vi "Main.vi"() -> ()   [LabVIEW 2017]
doc: "Use this template to build a simple state machine design pattern. Each state executes code and determines which state to transition to."
uses:
  <vilib>/robotics/Controls/Compass Indicator/Compass Indicator.xctl
  controls/State.ctl
  controls/Data.ctl
  <vilib>/Instr/_visa.llb/VISA Configure Serial Port (Instr).vi
  support/VariaveisGlobais.vi
panel:
  out "DadosGPS":dbl[][](array[numeric])
  in  "Controles":T1(tab)
  out "Corrente de Saída":dbl caption="Numeric"
  out "SOC":dbl(slide)=100.0 scale=0.0..100.0
  out "Volt(V)":dbl(knob)=54.0 caption="Gauge" scale=0.0..60.0
  out "Velocidade do Barco":dbl(knob)=30.0 caption="Gauge" scale=0.0..50.0
  out "Corrente de Entrada":dbl caption="Numeric"
  out "Longitude do Barco":dbl=-48.640396 format="%#.6g"
  out "Banco de Bateria":dbl[][](array[slide])=[[3.33, 3.33, 3.33, 3.33], [3.33, 3.33, 3.33, 3.33], [3.33, 3.33, 3.33, 3.33], [3.33, 3.33, 3.33, 3.33], [3.33, 3.33, 3.33, 3.33]] scale=0.0..5.0
  out "Voltagem Mínima":dbl=3.33
  out "Voltagem Máxima":dbl=3.33
  out "Sistema de Placa Solar":bool[][](array[boolean])
  in  "Color Box":u32(colorbox)=16777225
  out "Latitude do Barco":dbl=-26.244263 format="%#.6g"
  out "Latitude do Terra":dbl=-26.244263 format="%#.6g"
  out "Longitude do Terra":dbl=-48.640396 format="%#.6g"
  out "Compass Indicator":dbl(xcontrol)
  out "Distance to Destination km":dbl=0.005416306273989337
  out "Dados Recebidos":string
  out "PlotGeral":dbl[][](graph)
  out "Plotagem":dbl[](graph)
  in  "PlotarDados":u16(ring) caption="Ring" items=["Voltagem", "CorrenteE", "CorrenteS", "Velocidade"]
  out "Historico de Dados":string[][](table)
  in  "Intercalar":i32=1
  in  "N° Pontos":i32=5
  in  "Adionar Pontos":bool
  in  "WebBrowser":refnum<k7>(container)
  in  "Color":string(combo)
  in  "Size":string(combo)
  in  "Character":string(combo)
  in  "Latitude 2":dbl=-3.091948 format="%#.6g"
  in  "Longitude 2":dbl=-60.017863 format="%#.6g"
  in  "Zoom":sgl=16.0 format="%#.1g"
  in  "Size Y":dbl=650.0
  in  "Size X":dbl=450.0
  in  "Map Format":string(combo)="roadmap"
  in  "AtualizarMapa":bool
  in  "Dados no Arquivo":bool
  in  "Titulo do Arquivo":string="Telemetria-"
  in  "Inserir Data":bool=TRUE
  in  "Salvar":bool
  in  "Abrir":bool
  in  "Baud Rate":string(combo)="115200"
  in  "Porta COM":refnum<visa-resource-name>="COM4"
  in  "Data Bits":u16=8 caption="Numeric"
  in  "Parity":enum16{"None", "Odd", "Even", "Mark", "Space"}(ring)
  in  "Conectar":bool
  in  "Desconectar":bool
  in  "ByteCount":u32=100 caption="Numeric"
  out "ProgressoBarco":dbl(slide) scale=0.0..1.0
  in  "DesligarApp":bool
  in  "ResetButton":bool
  in  "Janela":T2(radio)
  in  "Cancel":bool
  in  "LerDados":bool
  # "Telemetria - Leviatã"
  # "Cargas"
  # "Banco de Baterias"
  # "Poraquê"
  # "Plotagem de Dados"
  # "Análise de Localização no Mapa"
  # "Dados de Telemetria"
  # "Configuração de Porta"
  # "Leviatã: Barco Poraquê\ntime de telemetria do barco a fim de realizar a leitura da bateria do barco\n\n\n\n\n\n\n\n\n\nDesenvolvido por: Alan Shishido / Igor Souza"
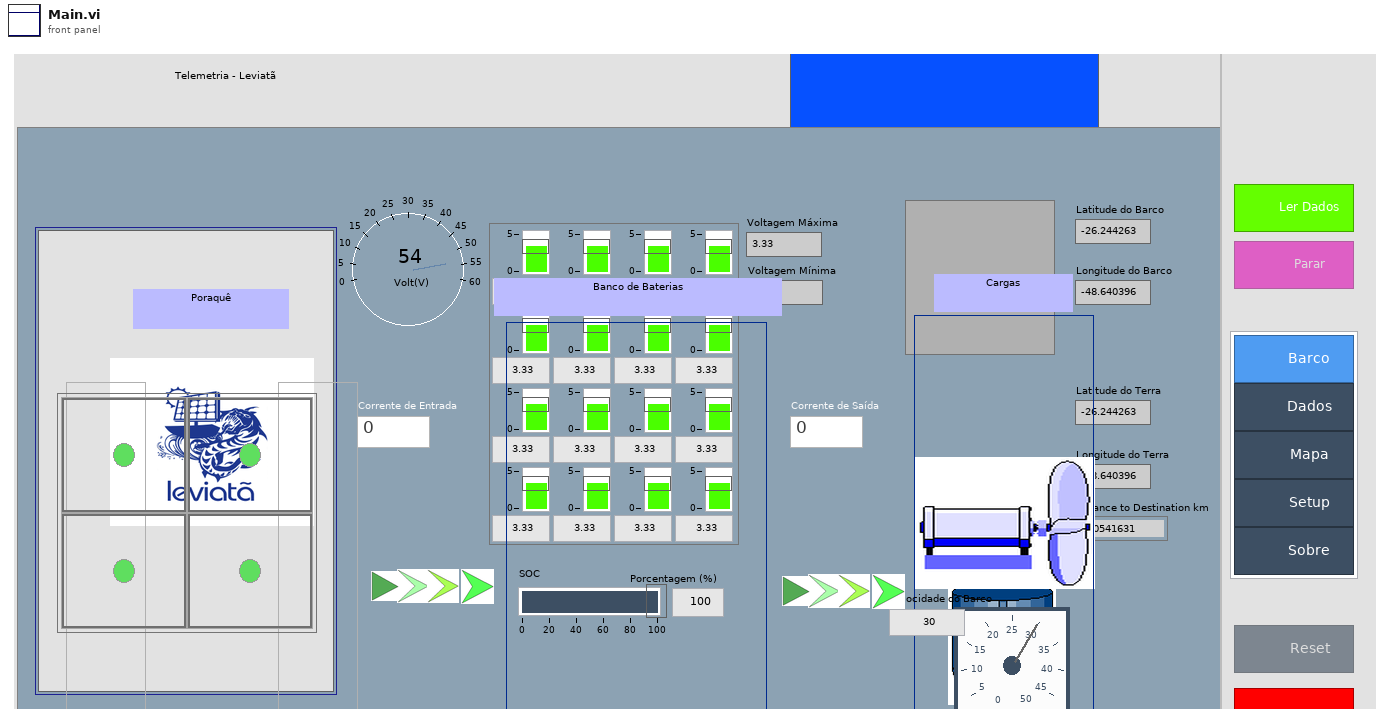
[diagram p1: front panel]
types:
  T1 = enum32{"Barco", "Gráfico", "Mapa", "Configuração", "Sobre"}
  T2 = enum32{"BarcoButton", "DadosButton", "MapaButton", "SetupButton", "SobreButton"}
  T3 = typedef "Data.ctl" = cluster{"PararOperação?":bool, "DadosSerial":string, "Dados 0":string, "Dados 1":string, "Dados 2":string, "Dados 3":string, "Dados 4":string, "Dados 5":string, "Dados 6":string, "Dados 7":string, "Dados 8":string, "Dados 9":string, "Dados 10":string, "Dados 11":string, "Dados 12":string, "Dados 13":string, "Dados 14":string, "Dados 15":string}
  T4 = cluster{"DadosBMS":T3, "SetupMapa":cluster{"Marker":string, "Path":string, "Markers Coordinates":string[][]}, "IteraçãoPrograma":cluster{"varBarco":i32, "varLerDados1":bool, "varLerDados2":bool, "varLerDados3":bool, "varLerDados4":bool}}
  T5 = typedef "State.ctl" = enum16{"Inicialização", "EsperaEvento", "bDesconectarSerial", "bConectar Serial", "bLerDadosSerial", "ProcessaDadosSerial", "AtualizaDadosSerial", "ArquivoDadosIncremental", "ClearAllDisplay", "AtualizarStaticMaps", "AdicionarPontosStaticMaps", "Sair"}
  T6 = enum8{"Enabled", "Disabled", "Disabled and Grayed Out"}
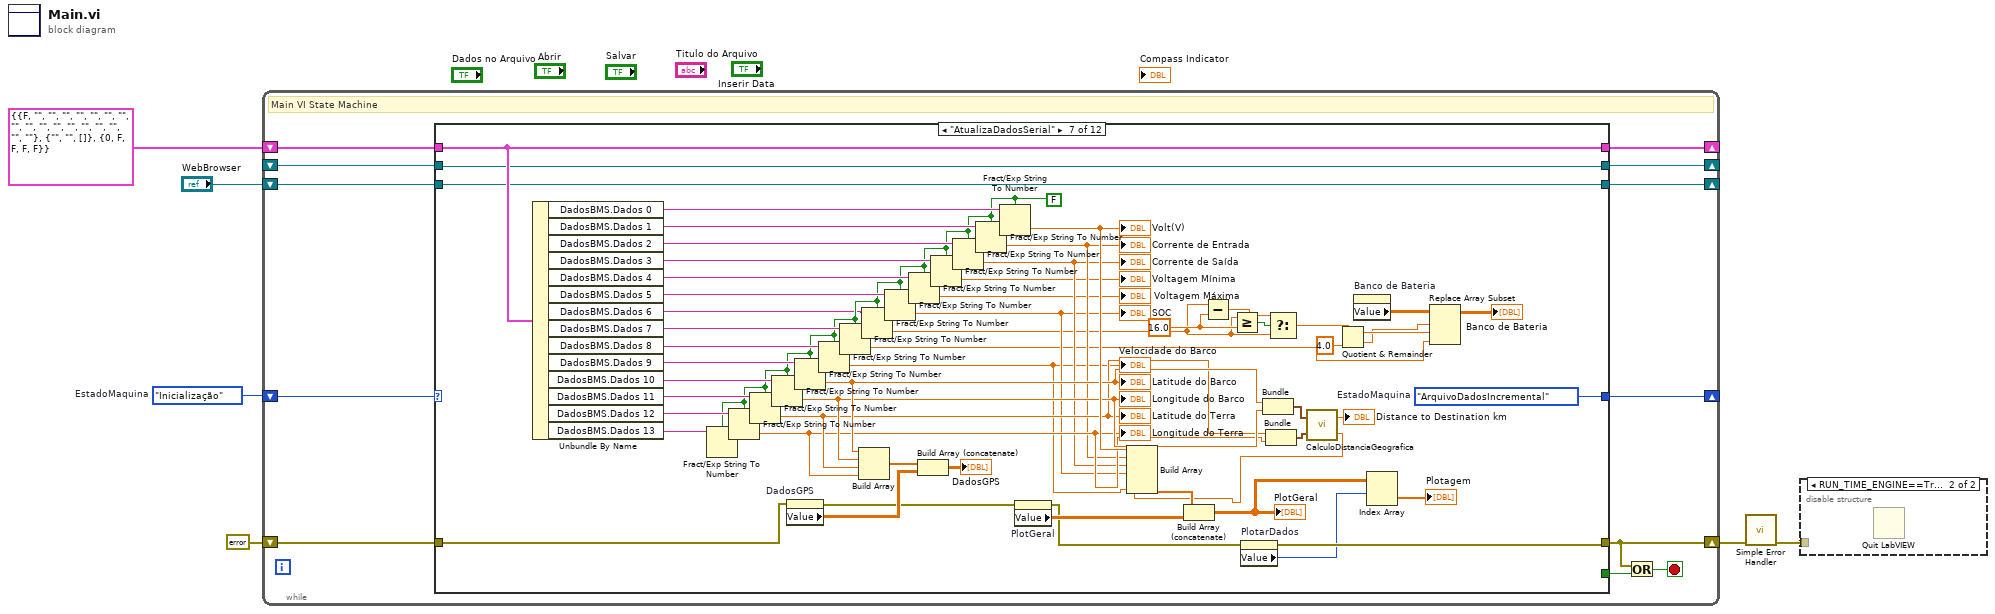
[diagram p0: block diagram]
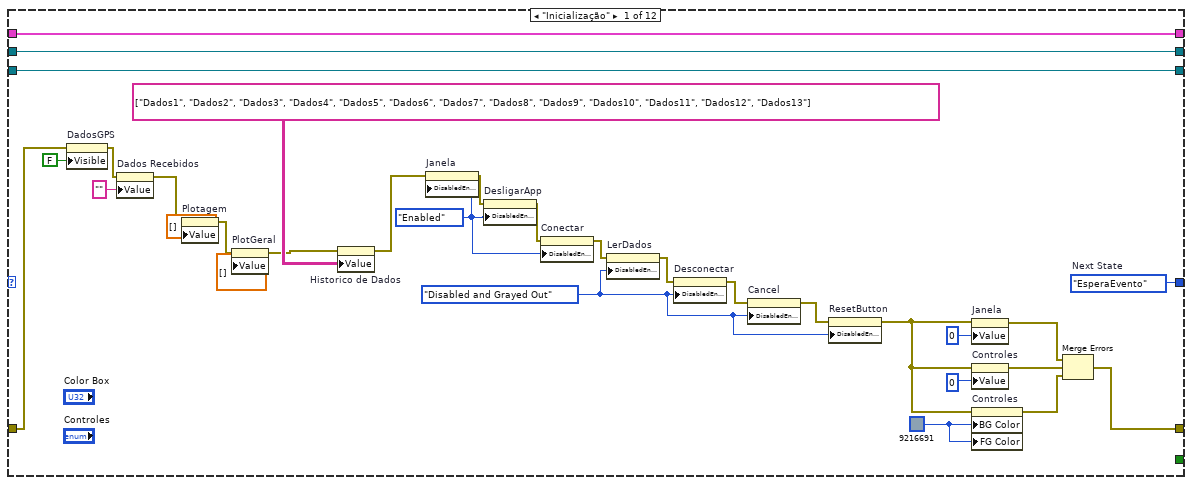
[diagram p2: hidden frame]
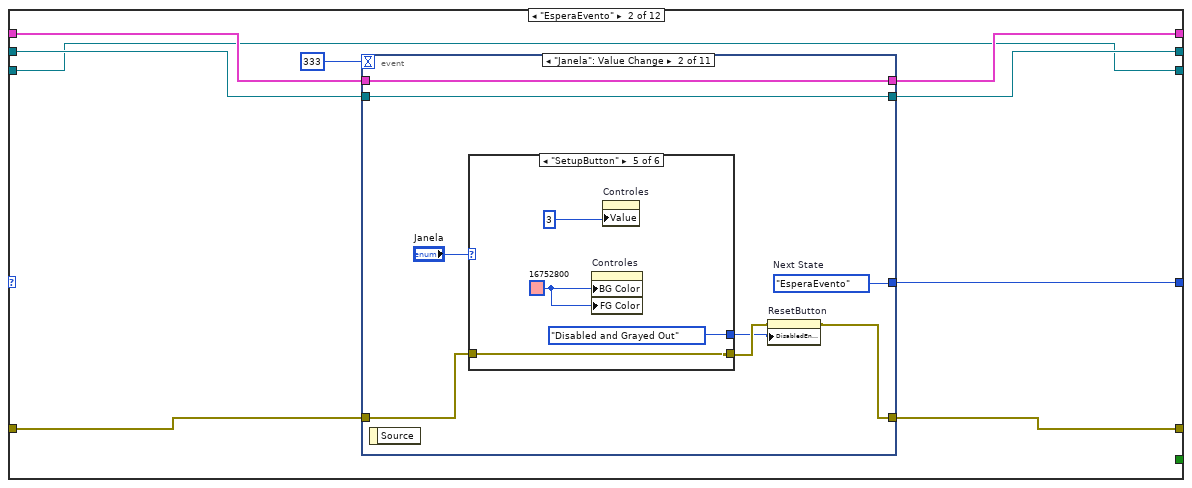
[diagram p3: hidden frame]
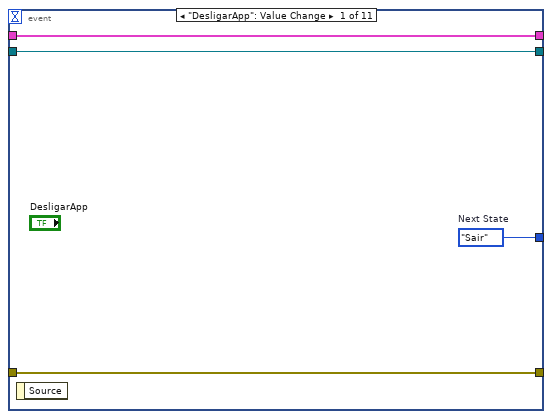
[diagram p4: hidden frame]
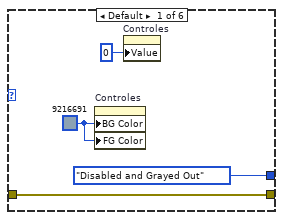
[diagram p5: hidden frame]
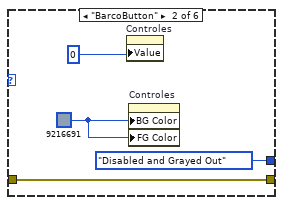
[diagram p6: hidden frame]
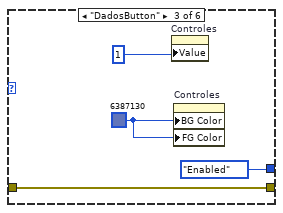
[diagram p7: hidden frame]
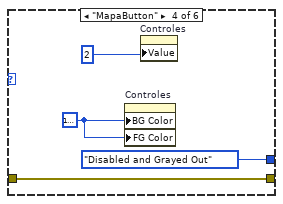
[diagram p8: hidden frame]
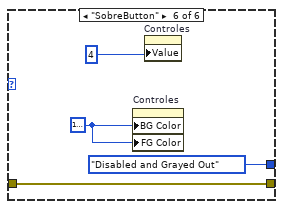
[diagram p9: hidden frame]
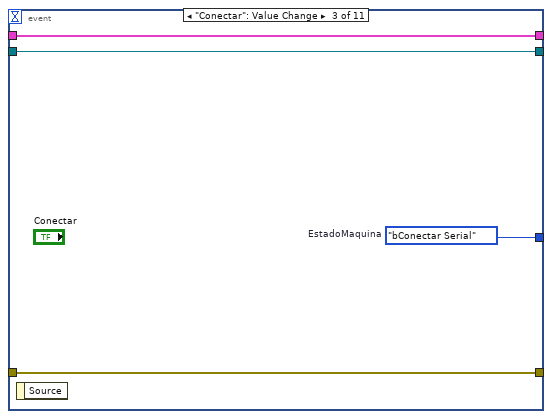
[diagram p10: hidden frame]
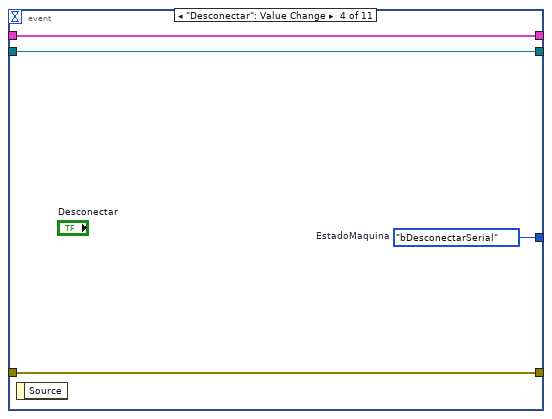
[diagram p11: hidden frame]
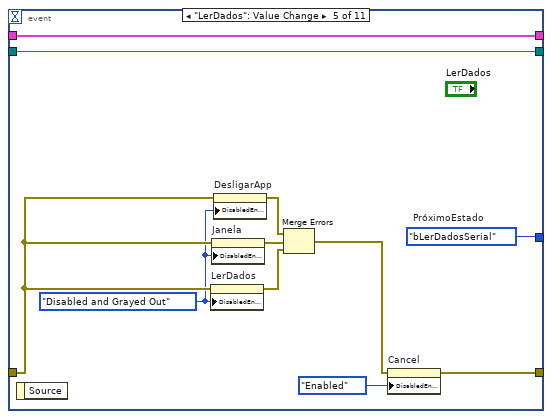
[diagram p12: hidden frame]
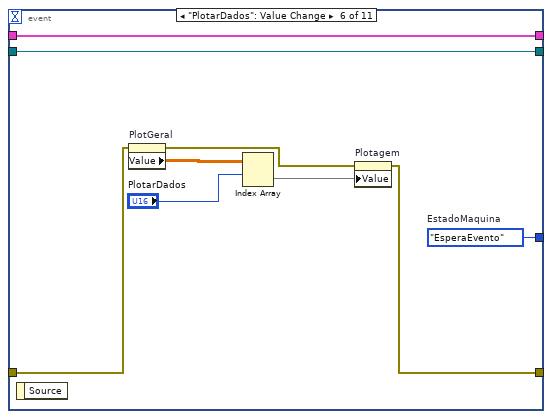
[diagram p13: hidden frame]
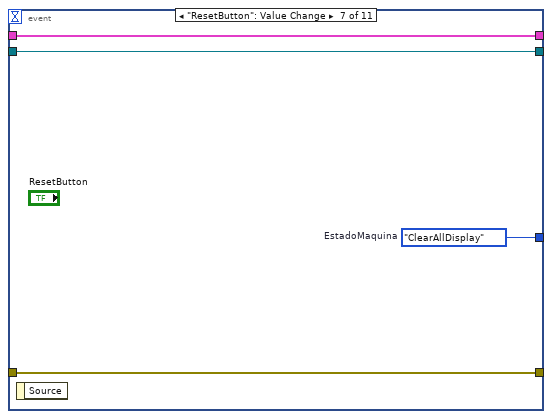
[diagram p14: hidden frame]
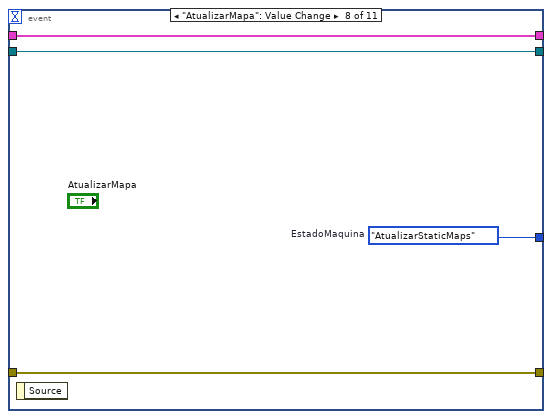
[diagram p15: hidden frame]
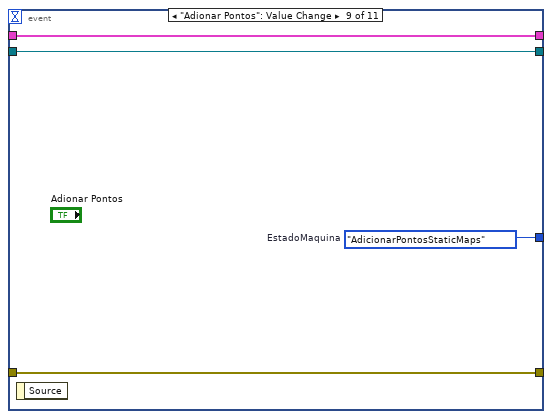
[diagram p16: hidden frame]
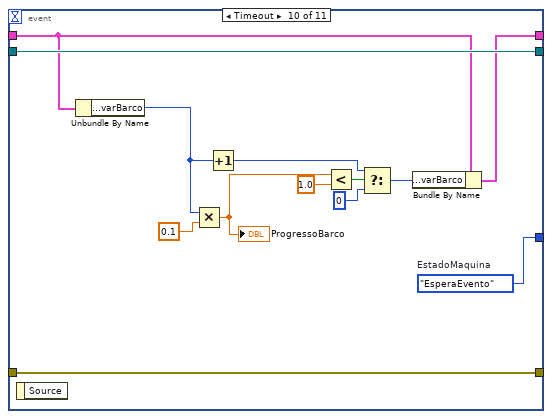
[diagram p17: hidden frame]
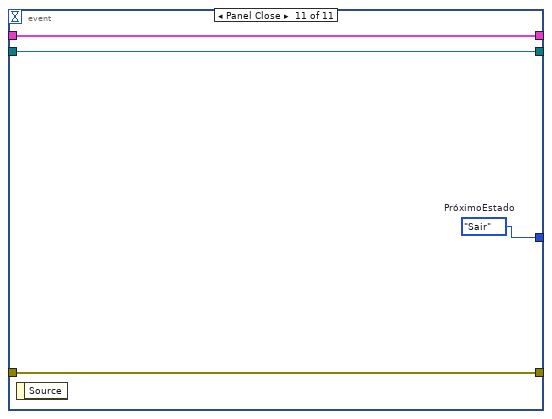
[diagram p18: hidden frame]
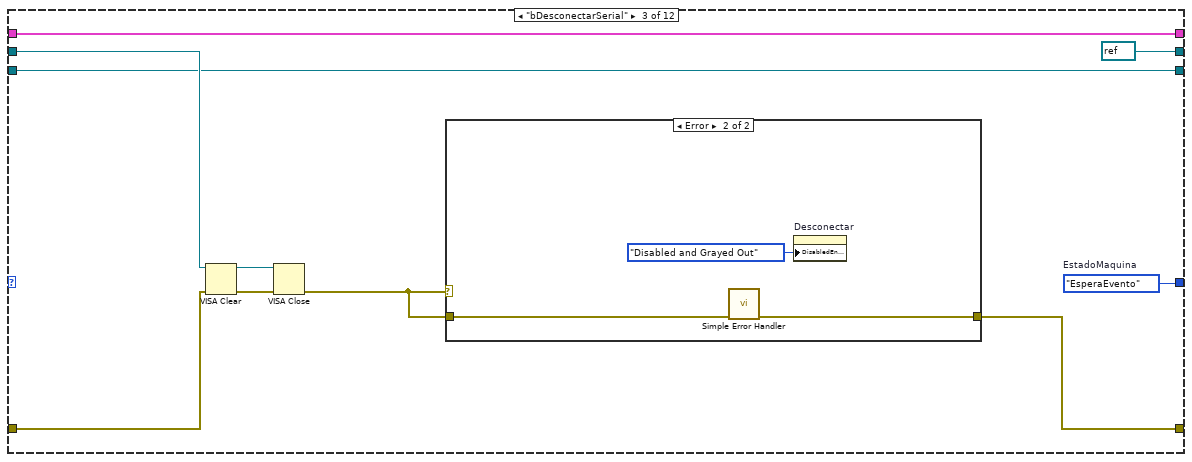
[diagram p19: hidden frame]
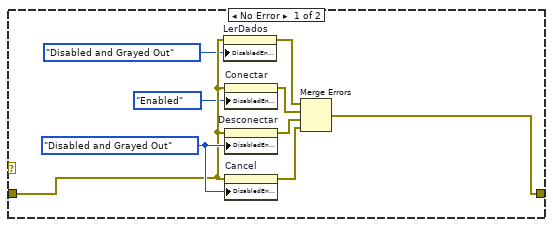
[diagram p20: hidden frame]
diagram:
  w6 = State."Inicialização"  # EstadoMaquina
  n1 = while {
    shift-right: [w17] -> _
    shift-left: w6 -> [w18]
    shift-right: [w15] -> _
    shift-left: T4 {"DadosBMS"={"PararOperação?"=FALSE, "DadosSerial"="", "Dados 0"="", "Dados 1"="", "Dados 2"="", "Dados 3"="", "Dados 4"="", "Dados 5"="", "Dados 6"="", "Dados 7"="", "Dados 8"="", "Dados 9"="", "Dados 10"="", "Dados 11"="", "Dados 12"="", "Dados 13"="", "Dados 14"="", "Dados 15"=""}, "SetupMapa"={"Marker"="", "Path"="", "Markers Coordinates"=[]}, "IteraçãoPrograma"={"varBarco"=0, "varLerDados1"=FALSE, "varLerDados2"=FALSE, "varLerDados3"=FALSE, "varLerDados4"=FALSE}} -> [w16]
    shift-right: [w11] -> w4
    shift-left: errorcluster {"status"=FALSE, "code"=0, "source"=""} ("error constant") -> [w14]
    shift-right: [w10] -> _
    shift-left: _ -> [w9]
    shift-right: [w7] -> _
    shift-left: "WebBrowser" -> [w8]
    stop <- w12 stop-if-true
    # "Main VI State Machine"
    n2 = case shown="\"AtualizaDadosSerial\"" w18 {
      tunnel: [w49 w58 w160 w191 w235 w273 w414 w455 w466 w490 w500 w535] -> w17
      tunnel: [_ _ _ _ _ _ _ _ _ _ _ w533] -> w13
      tunnel: w16 -> [w43 w57 w161 w192 w237 w268 w416 w421 w468 w479 w499 w534]
      tunnel: [w43 w56 w161 w192 w236 w267 w416 w420 w468 w479 w498 w534] -> w15
      tunnel: w14 -> [w26 w55 w158 w190 w238 w277 w386 w452 w458 w470 w502 w530]
      tunnel: [w32 w54 w155 w185 w222 w277 w384 w451 w457 w476 w502 errorcluster {"status"=FALSE, "code"=0, "source"=""} ("error constant")] -> w11
      tunnel: [w48 w52 refnum<visa-resource-name> refnum ("VISA resource name out") w184 w227 w276 w415 w418 w467 w491 w501 refnum<visa-resource-name> refnum ("VISA resource name out")] -> w10
      tunnel: w9 -> [w48 w51 w159 _ w239 w276 w415 w418 w467 w491 w501 w532]
      tunnel: w8 -> [w44 w50 w153 w175 w224 w257 w397 w419 w465 w478 w493 w527]
      tunnel: [w44 w50 w153 w175 w224 w257 w397 w419 w465 w477 w493 refnum<k7> refnum ("WebBrowser")] -> w7
      frame "Inicialização" {
        w47 = u32 9216691 ("Background Iterativa")
        w24 = T6."Disabled and Grayed Out" ("Disabled")
        w19 = T6."Enabled" ("Disabled")
        w49 = State."EsperaEvento"  # Next State
        # "Initialize - Initialize the application."
        n3 = property on="DadosGPS" class="Arr (strict)"(error in=w26, "Visible"=FALSE) -> (error out=w25:errorcluster)  [unwired: 1 in, 1 out]
        n4 = property on="Dados Recebidos" class="Str"(error in=w25, "Value"="" ("Dados Recebidos")) -> (error out=w38:errorcluster)  [unwired: 1 in, 1 out]
        n5 = property on="Plotagem" class="WFGraph (strict)"(error in=w38, "Value"=dbl[] [] ("Plotagem")) -> (error out=w37:errorcluster)  [unwired: 1 in, 1 out]
        n6 = property on="PlotGeral" class="WFGraph (strict)"(error in=w37, "Value"=dbl[][] [] ("Plotagem 2")) -> (error out=w36:errorcluster)  [unwired: 1 in, 1 out]
        n7 = property on="Historico de Dados" class="Tbl (strict)"(error in=w36, "Value"=string[][] [["Dados1", "Dados2", "Dados3", "Dados4", "Dados5", "Dados6", "Dados7", "Dados8", "Dados9", "Dados10", "Dados11", "Dados12", "Dados13"]] ("Historico de Dados")) -> (error out=w28:errorcluster)  [unwired: 1 in, 1 out]
        n8 = property on="Janela" class="RadioBtnsControl (strict)"(error in=w28, "DisabledEnum"=w19) -> (error out=w20:errorcluster)  [unwired: 1 in, 1 out]
        n9 = property on="DesligarApp" class="Bool"(error in=w20, "DisabledEnum"=w19) -> (error out=w21:errorcluster)  [unwired: 1 in, 1 out]
        n10 = property on="Conectar" class="Bool"(error in=w21, "DisabledEnum"=w19) -> (error out=w29:errorcluster)  [unwired: 1 in, 1 out]
        n11 = property on="LerDados" class="Bool"(error in=w29, "DisabledEnum"=w24) -> (error out=w30:errorcluster)  [unwired: 1 in, 1 out]
        n12 = property on="Desconectar" class="Bool"(error in=w30, "DisabledEnum"=w24) -> (error out=w39:errorcluster)  [unwired: 1 in, 1 out]
        n13 = property on="Cancel" class="Bool"(error in=w39, "DisabledEnum"=w24) -> (error out=w23:errorcluster)  [unwired: 1 in, 1 out]
        n14 = property on="ResetButton" class="Bool"(error in=w23, "DisabledEnum"=w24) -> (error out=w22:errorcluster)  [unwired: 1 in, 1 out]
        n15 = property on="Janela" class="RadioBtnsControl (strict)"(error in=w22, "Value"=0) -> (error out=w33:errorcluster)  [unwired: 1 in, 1 out]
        n16 = property on="Controles" class="TabCtl (strict)"(error in=w22, "Value"=0) -> (error out=w35:errorcluster)  [unwired: 1 in, 1 out]
        n17 = property on="Controles" class="TabCtl (strict)"(error in=w22, "BG Color"=w47, "FG Color"=w47) -> (error out=w34:errorcluster)  [unwired: 1 in, 1 out]
        n18 = Merge Errors(w33, w35, w34) -> (w32:errorcluster)
      }
      frame "EsperaEvento" {
        # "Wait for Event - Use an Event Structure to monitor the user interface for events that run different states of the state machine."
        n19 = event shown="[1] \"Janela\": Value Change" {
          selector: _ -> [_ _ _ _ _ _ _ _ _ _ _]
          dyn-events: _ -> [_ _ _ _ _ _ _ _ _ _ _]
          timeout: 333 -> [_ _ _ _ _ _ _ _ _ _ _]
          tunnel: [w62 w68 w96 w99 w111 w120 w123 w128 w131 w145 w148] -> w58
          tunnel: w57 -> [w61 w70 w98 w102 w113 w122 w126 w130 w134 w136 w151]
          tunnel: [w61 w70 w98 w102 w113 w122 w126 w130 w134 w135 w151] -> w56
          tunnel: w55 -> [w60 w66 w97 w101 w105 w115 w125 w129 w133 w147 w150]
          tunnel: [w60 w65 w97 w101 w109 w114 w125 w129 w133 w147 w150] -> w54
          tunnel: [w59 w67 w95 w100 w112 w121 w124 w127 w132 w139 w149] -> w52
          tunnel: w51 -> [w59 w67 w95 w100 w112 w121 w124 w127 w132 w139 w149]
          event "DesligarApp": Value Change {
            w62 = State."Sair"  # Next State
            n20 = event-data() -> ()  [unwired: 1 in, 1 out]
          }
          event "Janela": Value Change {
            w68 = State."EsperaEvento"  # Next State
            n21 = event-data() -> ()  [unwired: 1 in, 1 out]
            n22 = case shown="\"SetupButton\"" "Janela" {
              tunnel: [T6."Disabled and Grayed Out" ("Disabled") T6."Disabled and Grayed Out" ("Disabled") T6."Enabled" ("Disabled") T6."Disabled and Grayed Out" ("Disabled") T6."Disabled and Grayed Out" ("Disabled") T6."Disabled and Grayed Out" ("Disabled")] -> w63
              tunnel: [w71 w76 w80 w84 w88 w92] -> w64
              tunnel: w66 -> [w71 w76 w80 w84 w88 w92]
              frame Default {
                w74 = u32 9216691 ("Background Iterativa")
                n23 = property on="Controles" class="TabCtl (strict)"("BG Color"=w74, "FG Color"=w74) -> ()  [unwired: 2 in, 2 out]
                n24 = property on="Controles" class="TabCtl (strict)"("Value"=0) -> ()  [unwired: 2 in, 2 out]
              }
              frame "BarcoButton" {
                w77 = u32 9216691 ("Background Iterativa")
                n25 = property on="Controles" class="TabCtl (strict)"("Value"=0) -> ()  [unwired: 2 in, 2 out]
                n26 = property on="Controles" class="TabCtl (strict)"("BG Color"=w77, "FG Color"=w77) -> ()  [unwired: 2 in, 2 out]
              }
              frame "DadosButton" {
                w81 = u32 6387130 ("Background Iterativa")
                n27 = property on="Controles" class="TabCtl (strict)"("Value"=1) -> ()  [unwired: 2 in, 2 out]
                n28 = property on="Controles" class="TabCtl (strict)"("BG Color"=w81, "FG Color"=w81) -> ()  [unwired: 2 in, 2 out]
              }
              frame "MapaButton" {
                w86 = u32 16777216 ("Background Iterativa")
                n29 = property on="Controles" class="TabCtl (strict)"("BG Color"=w86, "FG Color"=w86) -> ()  [unwired: 2 in, 2 out]
                n30 = property on="Controles" class="TabCtl (strict)"("Value"=2) -> ()  [unwired: 2 in, 2 out]
              }
              frame "SetupButton" {
                w90 = u32 16752800 ("Background Iterativa")
                n31 = property on="Controles" class="TabCtl (strict)"("BG Color"=w90, "FG Color"=w90) -> ()  [unwired: 2 in, 2 out]
                n32 = property on="Controles" class="TabCtl (strict)"("Value"=3) -> ()  [unwired: 2 in, 2 out]
              }
              frame "SobreButton" {
                w94 = u32 16777226 ("Background Iterativa")
                n33 = property on="Controles" class="TabCtl (strict)"("BG Color"=w94, "FG Color"=w94) -> ()  [unwired: 2 in, 2 out]
                n34 = property on="Controles" class="TabCtl (strict)"("Value"=4) -> ()  [unwired: 2 in, 2 out]
              }
            }
            n35 = property on="ResetButton" class="Bool"(error in=w64, "DisabledEnum"=w63) -> (error out=w65:errorcluster)  [unwired: 1 in, 1 out]
          }
          event "Conectar": Value Change {
            w96 = State."bConectar Serial"  # EstadoMaquina
            n36 = event-data() -> ()  [unwired: 1 in, 1 out]
          }
          event "Desconectar": Value Change {
            w99 = State."bDesconectarSerial"  # EstadoMaquina
            n37 = event-data() -> ()  [unwired: 1 in, 1 out]
          }
          event "LerDados": Value Change {
            w103 = T6."Disabled and Grayed Out" ("Disabled")
            w111 = State."bLerDadosSerial"  # PróximoEstado
            n38 = event-data() -> ()  [unwired: 1 in, 1 out]
            n39 = property on="LerDados" class="Bool"(error in=w105, "DisabledEnum"=w103) -> (error out=w106:errorcluster)  [unwired: 1 in, 1 out]
            n40 = property on="Janela" class="RadioBtnsControl (strict)"(error in=w105, "DisabledEnum"=w103) -> (error out=w108:errorcluster)  [unwired: 1 in, 1 out]
            n41 = property on="DesligarApp" class="Bool"(error in=w105, "DisabledEnum"=w103) -> (error out=w104:errorcluster)  [unwired: 1 in, 1 out]
            n42 = Merge Errors(w104, w108, w106) -> (w107:errorcluster)
            n43 = property on="Cancel" class="Bool"(error in=w107, "DisabledEnum"=T6."Enabled" ("Disabled")) -> (error out=w109:errorcluster)  [unwired: 1 in, 1 out]
          }
          event "PlotarDados": Value Change {
            w120 = State."EsperaEvento"  # EstadoMaquina
            n44 = event-data() -> ()  [unwired: 1 in, 1 out]
            n45 = property on="PlotGeral" class="WFGraph (strict)"(error in=w115) -> (error out=w116:errorcluster, "Value"=w119:dbl[][])  [unwired: 1 in, 1 out]
            n46 = Index Array(array=w119, index (row)="PlotarDados") -> (element=w117:dbl[])  [unwired: 1 in]
            n47 = property on="Plotagem" class="WFGraph (strict)"(error in=w116, "Value"=w117) -> (error out=w114:errorcluster)  [unwired: 1 in, 1 out]
          }
          event "ResetButton": Value Change {
            w123 = State."ClearAllDisplay"  # EstadoMaquina
            n48 = event-data() -> ()  [unwired: 1 in, 1 out]
          }
          event "AtualizarMapa": Value Change {
            w128 = State."AtualizarStaticMaps"  # EstadoMaquina
            n49 = event-data() -> ()  [unwired: 1 in, 1 out]
          }
          event "Adionar Pontos": Value Change {
            w131 = State."AdicionarPontosStaticMaps"  # EstadoMaquina
            n50 = event-data() -> ()  [unwired: 1 in, 1 out]
          }
          event Timeout {
            w145 = State."EsperaEvento"  # EstadoMaquina
            n51 = event-data() -> ()  [unwired: 1 in, 1 out]
            n52 = Unbundle By Name(w136) -> ("IteraçãoPrograma.varBarco"=w137:i32)
            n53 = Multiply(x=w137, y=0.1) -> (x*y=w140:dbl)
            "ProgressoBarco" <- w140
            n54 = Increment(x=w137) -> (x+1=w142:i32)
            n55 = Less?(x=w140, y=1.0) -> (x < y?=w143:bool)
            n56 = Select(t=w142, s=w143, f=0) -> (s? t:f=w138:i32)
            n57 = Bundle By Name(cluster=w136, "IteraçãoPrograma.varBarco"=w138) -> (w135:T4)
          }
          event Panel Close {
            w148 = State."Sair"  # PróximoEstado
            n58 = event-data() -> ()  [unwired: 1 in, 1 out]
          }
        }
      }
      frame "bDesconectarSerial" {
        w160 = State."EsperaEvento"  # EstadoMaquina
        n59 = VISA Clear(VISA resource name=w159, error in (no error)=w158) -> (VISA resource name out=w157:refnum<visa-resource-name>, error out=w156:errorcluster)
        n60 = VISA Close(VISA resource name=w157, error in (no error)=w156) -> (error out=w152:errorcluster)
        n61 = case shown="Error" w152 {
          tunnel: w152 -> [w164 w173]
          tunnel: [w170 w172] -> w155
          frame No Error {
            w165 = T6."Disabled and Grayed Out" ("Disabled")
            n62 = property on="LerDados" class="Bool"(error in=w164, "DisabledEnum"=T6."Disabled and Grayed Out" ("Disabled")) -> (error out=w166:errorcluster)  [unwired: 1 in, 1 out]
            n63 = property on="Conectar" class="Bool"(error in=w164, "DisabledEnum"=T6."Enabled" ("Disabled")) -> (error out=w167:errorcluster)  [unwired: 1 in, 1 out]
            n64 = property on="Desconectar" class="Bool"(error in=w164, "DisabledEnum"=w165) -> (error out=w168:errorcluster)  [unwired: 1 in, 1 out]
            n65 = property on="Cancel" class="Bool"(error in=w164, "DisabledEnum"=w165) -> (error out=w169:errorcluster)  [unwired: 1 in, 1 out]
            n66 = Merge Errors(w166, w167, w168, w169) -> (w170:errorcluster)
          }
          frame Error {
            n67 = call <vilib>:"Simple Error Handler.vi"("error in (no error)"=w173) -> ("error out"=w172:errorcluster)  [unwired: 4 in, 4 out]
            n68 = property on="Desconectar" class="Bool"("DisabledEnum"=T6."Disabled and Grayed Out" ("Disabled")) -> ()  [unwired: 2 in, 2 out]
          }
        }
      }
      frame "bConectar Serial" {
        w191 = State."EsperaEvento"  # EstadoMaquina
        n69 = Decimal String To Number(string="Baud Rate", default (0L)=u32 0 ("number")) -> (number=w178:u32)  [unwired: 1 in, 1 out]
        n70 = call-poly "VISA Configure Serial Port"("VISA resource name"="Porta COM", "timeout (10sec)"=u32 30000, "baud rate (9600)"=w178, "data bits (8)"="Data Bits", "parity (0:none)"=enum16{"None", "Odd", "Even", "Mark", "Space"}."None", "error in (no error)"=w190) -> ("VISA resource name out"=w187:refnum<visa-resource-name>, "error out"=w189:errorcluster)  [unwired: 8 in]
        n71 = Variant To Data(type="", Variant="Porta COM") -> (data=w182:string)  [unwired: 1 in, 1 out]
        n72 = VISA Open(error in (no error)=w189, VISA resource name=w187) -> (VISA resource name=w186:refnum<visa-resource-name>, error out=w188:errorcluster)  [unwired: 3 in]
        n73 = case shown="No Error" w188 {
          selector: w188 -> [w206 w215]
          tunnel: [w199 errorcluster {"status"=FALSE, "code"=0, "source"=""} ("error constant")] -> w185
          tunnel: w186 -> [w213 w216]
          tunnel: [w213 w216] -> w184
          tunnel: w182 -> [w212 _]
          frame No Error {
            w207 = u32 9216691 ("Background Iterativa")
            n74 = Concatenate Strings("Conectado: " ("message"), w212) -> (w211:string)
            n75 = property on="LerDados" class="Bool"(error in=w206, "DisabledEnum"=T6."Enabled" ("Disabled")) -> (error out=w204:errorcluster)  [unwired: 1 in, 1 out]
            n76 = property on="Conectar" class="Bool"(error in=w206, "DisabledEnum"=T6."Disabled and Grayed Out" ("Disabled")) -> (error out=w203:errorcluster)  [unwired: 1 in, 1 out]
            n77 = property on="Desconectar" class="Bool"(error in=w206, "DisabledEnum"=T6."Enabled" ("Disabled")) -> (error out=w202:errorcluster)  [unwired: 1 in, 1 out]
            n78 = property on="Cancel" class="Bool"(error in=w206, "DisabledEnum"=T6."Disabled and Grayed Out" ("Disabled")) -> (error out=w201:errorcluster)  [unwired: 1 in, 1 out]
            n79 = Merge Errors(w204, w203, w202, w201) -> (w197:errorcluster)
            n80 = One Button Dialog(message=w211, button name ("OK")="Continuar") -> ()  [unwired: 1 out]
            n81 = property on="Controles" class="TabCtl (strict)"(error in=w197, "BG Color"=w207, "FG Color"=w207) -> (error out=w198:errorcluster)  [unwired: 1 in, 1 out]
            n82 = property on="Janela" class="RadioBtnsControl (strict)"(error in=w197, "Value"=0) -> (error out=w195:errorcluster)  [unwired: 1 in, 1 out]
            n83 = property on="Controles" class="TabCtl (strict)"(error in=w197, "Value"=0) -> (error out=w200:errorcluster)  [unwired: 1 in, 1 out]
            n84 = Merge Errors(w195, w200, w198) -> (w199:errorcluster)
          }
          frame Error {
            n85 = call <vilib>:"Simple Error Handler.vi"("error in (no error)"=w215) -> ()  [unwired: 4 in, 5 out]
          }
        }
      }
      frame "bLerDadosSerial" {
        w234 = State."EsperaEvento"  # EstadoMaquina
        w233 = State."ProcessaDadosSerial"  # EstadoMaquina
        n86 = VISA Read(VISA resource name=w239, byte count="ByteCount", error in (no error)=w238) -> (VISA resource name out=w226:refnum<visa-resource-name>, read buffer=w225:string, error out=w228:errorcluster)  [unwired: 1 out]
        "Dados Recebidos" <- w225
        n87 = Bundle By Name(cluster=w237, "DadosBMS.DadosSerial"=w225) -> (w236:T4)
        n88 = VISA Clear(VISA resource name=w226, error in (no error)=w228) -> (VISA resource name out=w227:refnum<visa-resource-name>, error out=w229:errorcluster)
        n89 = Unbundle By Name(w229) -> ("code"=w231:i32)
        n90 = case shown="0, Default" w231 {
          tunnel: w229 -> [w250 _ _]
          tunnel: [w250 errorcluster {"status"=FALSE, "code"=0, "source"=""} ("error constant") errorcluster {"status"=FALSE, "code"=0, "source"=""} ("error constant")] -> w223
          tunnel: [FALSE w251 w254] -> w219
          frame 0, Default {
            n91 = global write "VariaveisGlobais.vi" "IndicesDados"(0 ("IndicesDados")) -> ()
          }
          frame -1073807346, -1073807253 {
            n92 = One Button Dialog(message="Erro: Serial não Conectado") -> (true=w251:bool)  [unwired: 1 in]
          }
          frame -1073807339 {
            n93 = One Button Dialog(message="Erro: Time Out") -> (true=w254:bool)  [unwired: 1 in]
          }
        }
        n94 = Or(x="Cancel", y=w219) -> (x .or. y?=w221:bool)
        n95 = case shown="False" w221 {
          selector: w221 -> [w241 w247]
          tunnel: [w241 w247] -> w218
          tunnel: w223 -> [w240 w243]
          tunnel: [w240 w245] -> w222
          frame False {
          }
          frame True {
            w242 = T6."Enabled" ("Disabled")
            n96 = property on="LerDados" class="Bool"(error in=w243, "DisabledEnum"=w242) -> (error out=w244:errorcluster)  [unwired: 1 in, 1 out]
            n97 = property on="Janela" class="RadioBtnsControl (strict)"(error in=w243, "DisabledEnum"=w242) -> ()  [unwired: 1 in, 2 out]
            n98 = property on="DesligarApp" class="Bool"(error in=w243, "DisabledEnum"=w242) -> ()  [unwired: 1 in, 2 out]
            n99 = property on="Cancel" class="Bool"(error in=w244, "DisabledEnum"=T6."Disabled and Grayed Out" ("Disabled")) -> (error out=w245:errorcluster)  [unwired: 1 in, 1 out]
          }
        }
        n100 = Select(t=w234, s=w218, f=w233) -> (s? t:f=w235:T5)
        n101 = Wait (ms)(milliseconds to wait=u32 250) -> ()  [unwired: 1 out]
      }
      frame "ProcessaDadosSerial" {
        w271 = State."ProcessaDadosSerial"  # PróximoEstado
        w272 = State."AtualizaDadosSerial"  # PróximoEstado
        n102 = Unbundle By Name(w268) -> ("DadosBMS.DadosSerial"=w275:string)
        n103 = Match Pattern(string=w275, regular expression=",") -> (before substring=w258:string, after substring=w264:string, offset past match=w270:i32)  [unwired: 1 in, 1 out]
        n104 = Equal?(x=w270, y=-1) -> (x = y?=w260:bool)
        n105 = global read "VariaveisGlobais.vi" "IndicesDados"() -> (w265:i32)
        n106 = case shown="4" w265 {
          tunnel: w258 -> [_ w282 w287 w292 w297 w302 w307 w312 w317 w322 w327 w332 w337 w342 w347 w352 w357]
          tunnel: w268 -> [w279 w284 w289 w294 w299 w304 w309 w314 w319 w324 w329 w334 w339 w344 w349 w354 w359]
          tunnel: [w279 w283 w288 w293 w298 w303 w308 w313 w318 w323 w328 w333 w338 w343 w348 w353 w358] -> w267
          tunnel: w264 -> [_ w281 w286 w291 w296 w301 w306 w311 w316 w321 w326 w331 w336 w341 w346 w351 w356]
          tunnel: [-1 ("IndicesDados") w280 w285 w290 w295 w300 w305 w310 w315 w320 w325 w330 w335 w340 w345 w350 w355] -> w263
          tunnel: w265 -> [_ w280 w285 w290 w295 w300 w305 w310 w315 w320 w325 w330 w335 w340 w345 w350 w355]
          frame Default {
          }
          frame 0 {
            n107 = Bundle By Name(cluster=w284, "DadosBMS.Dados 0"=w282, "DadosBMS.DadosSerial"=w281) -> (w283:T4)
          }
          frame 1 {
            n108 = Bundle By Name(cluster=w289, "DadosBMS.Dados 1"=w287, "DadosBMS.DadosSerial"=w286) -> (w288:T4)
          }
          frame 2 {
            n109 = Bundle By Name(cluster=w294, "DadosBMS.Dados 2"=w292, "DadosBMS.DadosSerial"=w291) -> (w293:T4)
          }
          frame 3 {
            n110 = Bundle By Name(cluster=w299, "DadosBMS.Dados 3"=w297, "DadosBMS.DadosSerial"=w296) -> (w298:T4)
          }
          frame 4 {
            n111 = Bundle By Name(cluster=w304, "DadosBMS.Dados 4"=w302, "DadosBMS.DadosSerial"=w301) -> (w303:T4)
          }
          frame 5 {
            n112 = Bundle By Name(cluster=w309, "DadosBMS.Dados 5"=w307, "DadosBMS.DadosSerial"=w306) -> (w308:T4)
          }
          frame 6 {
            n113 = Bundle By Name(cluster=w314, "DadosBMS.Dados 6"=w312, "DadosBMS.DadosSerial"=w311) -> (w313:T4)
          }
          frame 7 {
            n114 = Bundle By Name(cluster=w319, "DadosBMS.Dados 7"=w317, "DadosBMS.DadosSerial"=w316) -> (w318:T4)
          }
          frame 8 {
            n115 = Bundle By Name(cluster=w324, "DadosBMS.Dados 8"=w322, "DadosBMS.DadosSerial"=w321) -> (w323:T4)
          }
          frame 9 {
            n116 = Bundle By Name(cluster=w329, "DadosBMS.Dados 9"=w327, "DadosBMS.DadosSerial"=w326) -> (w328:T4)
          }
          frame 10 {
            n117 = Bundle By Name(cluster=w334, "DadosBMS.Dados 10"=w332, "DadosBMS.DadosSerial"=w331) -> (w333:T4)
          }
          frame 11 {
            n118 = Bundle By Name(cluster=w339, "DadosBMS.Dados 11"=w337, "DadosBMS.DadosSerial"=w336) -> (w338:T4)
          }
          frame 12 {
            n119 = Bundle By Name(cluster=w344, "DadosBMS.Dados 12"=w342, "DadosBMS.DadosSerial"=w341) -> (w343:T4)
          }
          frame 13 {
            n120 = Bundle By Name(cluster=w349, "DadosBMS.Dados 13"=w347, "DadosBMS.DadosSerial"=w346) -> (w348:T4)
          }
          frame 14 {
            n121 = Bundle By Name(cluster=w354, "DadosBMS.Dados 14"=w352, "DadosBMS.DadosSerial"=w351) -> (w353:T4)
          }
          frame 15 {
            n122 = Bundle By Name(cluster=w359, "DadosBMS.Dados 15"=w357, "DadosBMS.DadosSerial"=w356) -> (w358:T4)
          }
        }
        n123 = Increment(x=w263) -> (x+1=w266:i32)
        n124 = global write "VariaveisGlobais.vi" "IndicesDados"(w266) -> ()
        n125 = Equal?(x=w263, y=13) -> (x = y?=w261:bool)
        n126 = Or(x=w261, y=w260) -> (x .or. y?=w259:bool)
        n127 = Select(t=w272, s=w259, f=w271) -> (s? t:f=w273:T5)
      }
      frame "AtualizaDadosSerial" {
        w362 = 16.0 ("y")
        w371 = FALSE ("use system decimal point (T)")
        w414 = State."ArquivoDadosIncremental"  # EstadoMaquina
        n128 = Unbundle By Name(w416) -> ("DadosBMS.Dados 0"=w408:string, "DadosBMS.Dados 1"=w407:string, "DadosBMS.Dados 2"=w406:string, "DadosBMS.Dados 3"=w413:string, "DadosBMS.Dados 4"=w405:string, "DadosBMS.Dados 5"=w404:string, "DadosBMS.Dados 6"=w370:string, "DadosBMS.Dados 7"=w403:string, "DadosBMS.Dados 8"=w402:string, "DadosBMS.Dados 9"=w401:string, "DadosBMS.Dados 10"=w400:string, "DadosBMS.Dados 11"=w399:string, "DadosBMS.Dados 12"=w398:string, "DadosBMS.Dados 13"=w393:string)
        n129 = Fract/Exp String To Number(use system decimal point (T)=w371, string=w393) -> ()  [unwired: 2 in, 2 out]
        n130 = Fract/Exp String To Number(use system decimal point (T)=w371, string=w398) -> (number=w377:dbl)  [unwired: 2 in, 1 out]
        "Longitude do Terra" <- w377
        n131 = Fract/Exp String To Number(use system decimal point (T)=w371, string=w399) -> (number=w378:dbl)  [unwired: 2 in, 1 out]
        "Latitude do Terra" <- w378
        n132 = Fract/Exp String To Number(use system decimal point (T)=w371, string=w400) -> (number=w381:dbl)  [unwired: 2 in, 1 out]
        "Longitude do Barco" <- w381
        n133 = property on="DadosGPS" class="Arr (strict)"(error in=w386) -> (error out=w387:errorcluster, "Value"=w388:dbl[][])  [unwired: 1 in, 1 out]
        n134 = Fract/Exp String To Number(use system decimal point (T)=w371, string=w401) -> (number=w382:dbl)  [unwired: 2 in, 1 out]
        "Latitude do Barco" <- w382
        n135 = Fract/Exp String To Number(use system decimal point (T)=w371, string=w402) -> (number=w360:dbl)  [unwired: 2 in, 1 out]
        "Velocidade do Barco" <- w360
        n136 = Fract/Exp String To Number(use system decimal point (T)=w371, string=w403) -> (number=w368:dbl)  [unwired: 2 in, 1 out]
        n137 = Build Array(w382, w381, w378, w377) -> (w392:dbl[])
        n138 = Fract/Exp String To Number(use system decimal point (T)=w371, string=w370) -> (number=w361:dbl)  [unwired: 2 in, 1 out]
        n139 = Fract/Exp String To Number(use system decimal point (T)=w371, string=w404) -> (number=w369:dbl)  [unwired: 2 in, 1 out]
        "SOC" <- w369
        n140 = Fract/Exp String To Number(use system decimal point (T)=w371, string=w405) -> (number=→"Voltagem Máxima":dbl)  [unwired: 2 in, 1 out]
        n141 = Build Array (concatenate)(w392, w388) -> (→"DadosGPS":dbl[][])
        n142 = Fract/Exp String To Number(use system decimal point (T)=w371, string=w413) -> (number=→"Voltagem Mínima":dbl)  [unwired: 2 in, 1 out]
        n143 = Fract/Exp String To Number(use system decimal point (T)=w371, string=w406) -> (number=w374:dbl)  [unwired: 2 in, 1 out]
        "Corrente de Saída" <- w374
        n144 = Fract/Exp String To Number(use system decimal point (T)=w371, string=w407) -> (number=w375:dbl)  [unwired: 2 in, 1 out]
        "Corrente de Entrada" <- w375
        n145 = Fract/Exp String To Number(use system decimal point (T)=w371, string=w408) -> (number=w396:dbl)  [unwired: 2 in, 1 out]
        "Volt(V)" <- w396
        n146 = property on="PlotGeral" class="WFGraph (strict)"(error in=w387) -> (error out=w385:errorcluster, "Value"=w389:dbl[][])  [unwired: 1 in, 1 out]
        n147 = Subtract(x=w361, y=w362) -> (x-y=w363:dbl)
        n148 = Greater Or Equal?(x=w361, y=w362) -> (x >= y?=w365:bool)
        n149 = property on="PlotarDados" class="Ring (strict)"(error in=w385) -> (error out=w384:errorcluster, "Value"=w383:u16)  [unwired: 1 in, 1 out]
        n150 = Bundle(w382, w381) -> (w380:cluster{dbl, dbl})  [unwired: 1 in]
        n151 = Bundle(w378, w377) -> (w379:cluster{dbl, dbl})  [unwired: 1 in]
        n152 = Select(t=w363, s=w365, f=w361) -> (s? t:f=w364:dbl)
        n153 = call "CalculoDistanciaGeografica.vi"("Current Location (degrees)"=w379, "Destination (degrees)"=w380) -> ("Distance to Destination m"=w367:dbl, "Distance to Destination km"=→"Distance to Destination km":dbl)
        n154 = Build Array(w396, w375, w374, w369, w367, w360) -> (w395:dbl[])
        n155 = Build Array (concatenate)(w395, w389) -> (w390:dbl[][])
        "PlotGeral" <- w390
        n156 = Quotient & Remainder(x=w364, y=4.0) -> (x-y*floor(x/y)=w411:dbl, floor(x/y)=w410:dbl)
        n157 = property on="Banco de Bateria" class="Arr (strict)"() -> ("Value"=w412:dbl[][])  [unwired: 2 in, 2 out]
        n158 = Index Array(array=w390, index (row)=w383) -> (element=→"Plotagem":dbl[])  [unwired: 1 in]
        n159 = Replace Array Subset(array=w412, new element=w368, index (row)=w410, index (col)=w411) -> (→"Banco de Bateria":dbl[][])
      }
      frame "ArquivoDadosIncremental" {
        w455 = State."bLerDadosSerial"  # EstadoMaquina
        n160 = Unbundle By Name(w421) -> ("DadosBMS.Dados 0"=w449:string, "DadosBMS.Dados 1"=w448:string, "DadosBMS.Dados 2"=w447:string, "DadosBMS.Dados 3"=w446:string, "DadosBMS.Dados 4"=w445:string, "DadosBMS.Dados 5"=w444:string, "DadosBMS.Dados 6"=w443:string, "DadosBMS.Dados 7"=w442:string, "DadosBMS.Dados 8"=w441:string, "DadosBMS.Dados 9"=w440:string, "DadosBMS.Dados 10"=w439:string, "DadosBMS.Dados 11"=w438:string, "DadosBMS.Dados 12"=w437:string)
        n161 = property on="Historico de Dados" class="Tbl (strict)"(error in=w452) -> (error out=w451:errorcluster, "Value"=w453:string[][])  [unwired: 1 in, 1 out]
        n162 = Build Array(w449, w448, w447, w446, w445, w444, w443, w442, w441, w440, w439, w438, w437) -> (w454:string[])
        n163 = Insert Into Array(array=w453, index (row)=1, new element=w454) -> (→"Historico de Dados":string[][])  [unwired: 1 in]
        n164 = Unbundle By Name(w421) -> ("IteraçãoPrograma.varLerDados1"=w433:bool, "IteraçãoPrograma.varLerDados2"=w434:bool, "IteraçãoPrograma.varLerDados3"=w432:bool, "IteraçãoPrograma.varLerDados4"=w431:bool)
        n165 = Build Array(w433, w434, w432, w431) -> (w430:bool[])
        n166 = Boolean Array To Number(Boolean array=w430) -> (number=w435:u32)
        n167 = Increment(x=w435) -> (x+1=w436:u32)
        n168 = Number To Boolean Array(number=w436) -> (Boolean array=w429:bool[])
        n169 = Index Array(array=w429) -> (element #1=w425:bool, element #2=w422:bool, element #3=w423:bool, element #4=w424:bool)  [unwired: 4 in]
        n170 = Build Array(w425, w422) -> (w428:bool[])
        n171 = Build Array(w423, w424) -> (w427:bool[])
        n172 = Build Array(w428, w427) -> (→"Sistema de Placa Solar":bool[][])
        n173 = Bundle By Name(cluster=w421, "IteraçãoPrograma.varLerDados1"=w425, "IteraçãoPrograma.varLerDados2"=w422, "IteraçãoPrograma.varLerDados3"=w423, "IteraçãoPrograma.varLerDados4"=w424) -> (w420:T4)
      }
      frame "ClearAllDisplay" {
        w466 = State."EsperaEvento"  # PróximoEstado
        # "User State 2 - Replace this state with functionality for your own application."
        n174 = property on="Dados Recebidos" class="Str"(error in=w458, "Value"="" ("Dados Recebidos")) -> (error out=w463:errorcluster)  [unwired: 1 in, 1 out]
        n175 = property on="Plotagem" class="WFGraph (strict)"(error in=w463, "Value"=dbl[] [] ("Plotagem")) -> (error out=w462:errorcluster)  [unwired: 1 in, 1 out]
        n176 = property on="PlotGeral" class="WFGraph (strict)"(error in=w462, "Value"=dbl[][] [] ("Plotagem 2")) -> (error out=w459:errorcluster)  [unwired: 1 in, 1 out]
        n177 = property on="Historico de Dados" class="Tbl (strict)"(error in=w459, "Value"=string[][] [["Dados1", "Dados2", "Dados3", "Dados4", "Dados5", "Dados6", "Dados7", "Dados8", "Dados9", "Dados10", "Dados11", "Dados12", "Dados13"]] ("Historico de Dados")) -> (error out=w457:errorcluster)  [unwired: 1 in, 1 out]
      }
      frame "AtualizarStaticMaps" {
        w480 = "AIzaSyC0jIPNbLOk19LaEdHezqkIjEOWF-Yxd2E"  # Google Maps API Key
        w490 = State."EsperaEvento"  # EstadoMaquina
        # "This is an 86 character alphanumeric key supplied by Google"
        n178 = property on="DadosGPS" class="Arr (strict)"(error in=w470) -> (error out=w469:errorcluster, "Value"=w473:dbl[][])  [unwired: 1 in, 1 out]
        n179 = Index Array(array=w473, index (row)=0) -> (element=w474:dbl[])  [unwired: 1 in]
        n180 = Index Array(array=w474) -> (element #1=w472:dbl, element #2=w471:dbl)  [unwired: 2 in]
        n181 = Unbundle By Name(w479) -> ("SetupMapa.Marker"=w488:string, "SetupMapa.Path"=w489:string)
        n182 = call "Create Map URL.vi"("Map Format"="Map Format", "X"="Size X", "Lat"=w472, "Y"="Size Y", "Zoom"="Zoom", "Lon"=w471) -> ("String"=w486:string)  [unwired: 5 in]
        n183 = Concatenate Strings(w486, w488, w489, "&key=" ("string"), w480) -> (w487:string)
        n184 = invoke class="IWebBrowser2" method="Navigate"(reference=w478, error in=w469, "URL"=w487) -> (reference out=w477:refnum<k7>, error out=w476:errorcluster)  [unwired: 5 in, 6 out]
      }
      frame "AdicionarPontosStaticMaps" {
        w500 = State."AtualizarStaticMaps"  # EstadoMaquina
        n185 = Unbundle By Name(w499) -> ("SetupMapa.Marker"=w495:string, "SetupMapa.Markers Coordinates"=w497:string[][])
        n186 = for {
          N: "N° Pontos" -> [_]
          shift-right: [w516] -> w496
          shift-left: w497 -> [w517]
          shift-right: [w513] -> w494
          shift-left: w495 -> [w514]
          i -> [w505]
          w508 = "" ("Character")
          (unwired) 0 ("index (row)")
          n187 = property on="DadosGPS" class="Arr (strict)"() -> ("Value"=w512:dbl[][])  [unwired: 2 in, 2 out]
          n188 = Multiply(x=w505, y="Intercalar") -> (x*y=w504:i32)
          n189 = Index Array(array=w512, index (row)=w504) -> (element=w511:dbl[])  [unwired: 1 in]
          n190 = Index Array(array=w511) -> (element #1=w506:dbl, element #2=w507:dbl)  [unwired: 2 in]
          n191 = Number To Fractional String(number=w507) -> (F-format string=w523:string)  [unwired: 3 in]
          n192 = Number To Fractional String(number=w506) -> (F-format string=w524:string)  [unwired: 3 in]
          n193 = Concatenate Strings(w514, "&markers=color:", "orange" ("Color"), "%7Clabel:" ("string"), w508, "%7CSize:" ("string"), "tiny" ("Size"), "%7C" ("string"), w524, ",", w523) -> (w513:string)
          n194 = Build Array(w508, w523, w524) -> (w515:string[])
          n195 = Build Array (concatenate)(w517, w515) -> (w516:string[][])
        }
        n196 = Bundle By Name(cluster=w499, "SetupMapa.Marker"=w494, "SetupMapa.Markers Coordinates"=w496) -> (w498:T4)
      }
      frame "Sair" {
        w533 = TRUE  # Stop Loop?
        w535 = State."Sair"  # (Value Not Used)
        # "Exit - Exit the application."
        n197 = VISA Clear(VISA resource name=w532, error in (no error)=w530) -> (VISA resource name out=w529:refnum<visa-resource-name>, error out=w531:errorcluster)
        n198 = Close Reference(reference=w527) -> ()  [unwired: 1 in, 1 out]
        n199 = VISA Close(VISA resource name=w529, error in (no error)=w531) -> ()  [unwired: 1 out]
      }
    }
    n200 = Or(x=w11, y=w13) -> (x .or. y?=w12:bool)
  }
  n201 = call <vilib>:"Simple Error Handler.vi"("error in (no error)"=w4) -> ("error out"=w3:errorcluster)  [unwired: 4 in, 4 out]
  n202 = disable-structure shown="RUN_TIME_ENGINE==True" {
    disable-tunnel: w3 -> [_ _]
    frame condition #0 (active) {
    }
    frame condition #1 {
      n203 = Quit LabVIEW() -> ()  [unwired: 1 in]
    }
  }
